vi "Read Script Commands.vi"(7 "Test Name":string="IVIOKGD", 8 "Error In":errorcluster, 11 "All_Scripts":string[][](array[string])) -> (0 "Error Out":errorcluster, 1 "Script_Note":string[](array[string]), 2 "Script_Data":T2[](array[typedef]) {"Address" format="%.0x"}, 3 "Script_Functions":T1)   [LabVIEW 2013]
uses:
  Controls/Reg_Address_Data.ctl
  Controls/Script Functions_Array.ctl
  Controls/Script Functions.ctl
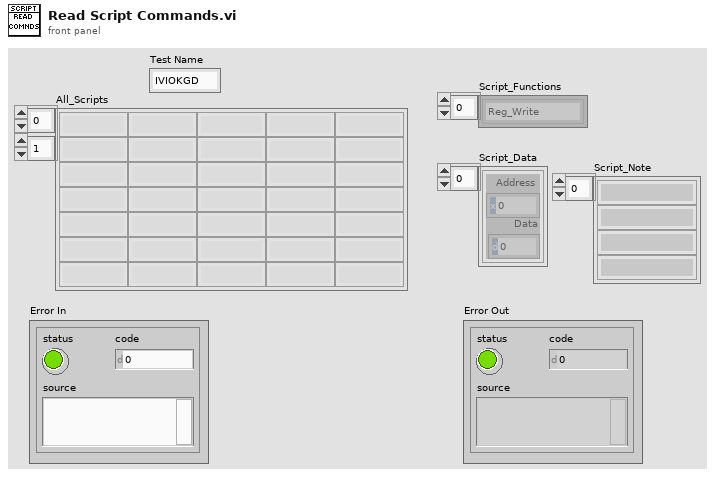
[diagram p1: front panel]
types:
  T1 = typedef "Script Functions_Array.ctl" = enum16{"Reg_Write", "Bit_Write", "Delay", "Read", "Measure"}[]
  T2 = typedef "Reg_Address_Data.ctl" = cluster{"Address":u8, "Data":u8}
  T3 = typedef "Script Functions.ctl" = enum16{"Reg_Write", "Bit_Write", "Delay", "Read", "Measure"}
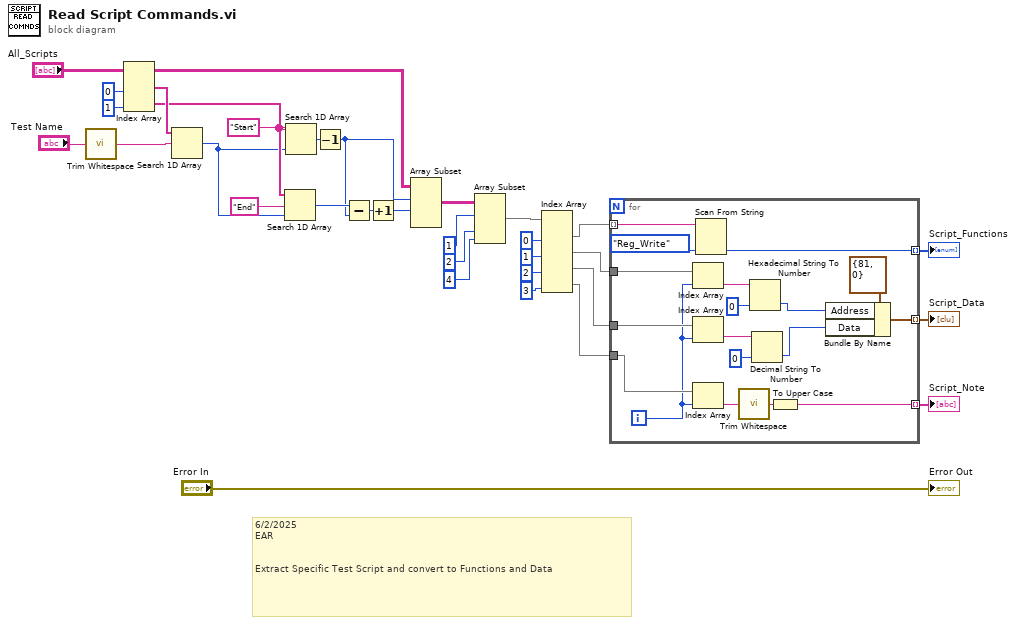
[diagram p0: block diagram]
diagram:
  # "6/2/2025\nEAR\n\n\nExtract Specific Test Script and convert to Functions and Data"
  n1 = call <vilib>:"Trim Whitespace.vi"("string"="Test Name") -> ("trimmed string"=w26:string)  [unwired: 1 in]
  n2 = Index Array(array="All_Scripts", index (col) #1=0 ("disabled index (col)"), index (col) #2=1 ("index (col)")) -> (element #1=w29:string[], element #2=w27:string[])  [unwired: 2 in]
  n3 = Search 1D Array(1D array=w29, element=w26) -> (index of element=w25:i32)  [unwired: 1 in]
  n4 = Search 1D Array(1D array=w27, element="End", start index (0)=w25) -> (index of element=w24:i32)
  n5 = Search 1D Array(1D array=w27, element="Start", start index (0)=w25) -> (index of element=w6:i32)
  n6 = Decrement(x=w6) -> (x-1=w4:i32)
  n7 = Subtract(x=w24, y=w4) -> (x-y=w23:i32)
  n8 = Increment(x=w23) -> (x+1=w5:i32)
  n9 = Array Subset(array="All_Scripts", index (row)=w4, length (row)=w5) -> (w22:string[][])  [unwired: 2 in]
  n10 = Array Subset(array=w22, index (row)=1 ("index"), index (col)=2 ("index"), length (col)=4 ("length")) -> (w15:string[][])  [unwired: 1 in]
  n11 = Index Array(array=w15, index (col) #1=0 ("disabled index (col)"), index (col) #2=1 ("index (col)"), index (col) #3=2 ("index (col)"), index (col) #4=3 ("index (col)")) -> (element #1=w12:string[], element #2=w11:string[], element #3=w10:string[], element #4=w2:string[])  [unwired: 4 in]
  n12 = for {
    tunnel: w12 -> [w49] mode=indexing
    tunnel: [w48] -> w7 mode=indexing
    tunnel: w11 -> [w47]
    tunnel: w10 -> [w46]
    tunnel: [w44] -> w9 mode=indexing
    tunnel: w2 -> [w37]
    tunnel: [w33] -> w1 mode=indexing
    i -> [w36]
    n13 = Index Array(array=w47, index=w36) -> (element=w43:string)
    n14 = Index Array(array=w46, index=w36) -> (element=w40:string)
    n15 = Index Array(array=w37, index=w36) -> (element=w35:string)
    n16 = Scan From String(input string=w49, default 1=Script_Functions."Reg_Write" ("Enum")) -> (output 1=w48:T3)  [unwired: 3 in, 3 out]
    n17 = call <vilib>:"Trim Whitespace.vi"("string"=w35) -> ("trimmed string"=w34:string)  [unwired: 1 in]
    n18 = Hexadecimal String To Number(string=w43, default (0uL)=u8 0 ("Address")) -> (number=w41:u8)  [unwired: 1 in, 1 out]
    n19 = Decimal String To Number(string=w40, default (0L)=u8 0 ("Address")) -> (number=w38:u8)  [unwired: 1 in, 1 out]
    n20 = To Upper Case(1:w34) -> (0:w33:string)
    n21 = Bundle By Name(cluster=T2 {"Address"=81, "Data"=0} ("Reg_Address_Data"), "Address"=w41, "Data"=w38) -> (w44:T2)
  }
  "Script_Data" <- w9
  "Script_Functions" <- w7
  "Script_Note" <- w1
  "Error Out" <- "Error In"
